vi "Main.vi"() -> ()   [LabVIEW 2025]
doc: "This simple VI control few elements of a Nikon Ti2 microscope.\nAny kind of supplementary element can be controlled with a new event type (flurorescence cube turret for example)"
uses:
  Controls/Presets.ctl
panel:
  in  "Step size (mm?)":dbl
  in  "Move Y+":bool
  in  "Move Y-":bool
  in  "Move X-":bool
  in  "Move X+":bool
  out "XY stage cluster":T1
  out "PFS cluster":T2
  in  "Presets":T3=2 items=["1- Bino - Brightfield"=1, "2- Bino - Fluo"=2, "3- Right - Brightfield"=3, "4- Right - Fluo"=4, "5- Left"=5]
  in  "Cluster commandes":T4={"Dia lamp"=TRUE, "Dia lamp intensity"=1689.1304347826087, "Objective"=2, "Light path"=2, "Z pos (µm)"=335593, "Filter wheel 2"=2, "Filter wheel 1"=2, "Shutter 2"=TRUE, "Shutter 1"=TRUE} {"Filter wheel 1" items=["1"=1, "2"=2, "3"=3, "4"=4, "5"=5, "6"=6]; "Filter wheel 2" items=["1"=1, "2"=2, "3"=3, "4"=4, "5"=5, "6"=6]; "Z pos (µm)" min=0 max=990000 step=100 scale=0.0..990000.0; "Light path" items=["1- Eyepiece"=1, "2- Right"=2, "3- Left + Eyepiece"=3, "4- Left"=4]; "Objective" items=["1- PLAN APO 100X 1,45 Oil"=1, "2- Empty"=2, "3- Empty"=3, "4- Empty"=4, "5- Empty"=5, "6- Empty"=6]; "Dia lamp intensity" scale=0.0..2100.0}
  out "Cluster µscope":T5
  in  "stop":bool
  in  "NikonTi2AxLib.INikonTi2AxMicroscope":refnum<k7>
  out "error out":errorcluster={"status"=TRUE, "code"=-9, "source"="Exception occured in Nikon.Ti2.Microscope.1: Failed in 231026_NikonTi2_Indicators_v2.vi"} caption="sortie d'erreur"
  in  "error in":errorcluster caption="entrée d'erreur"
  # "XY Stage"
  # "Perfect\nFocus\nSystem"
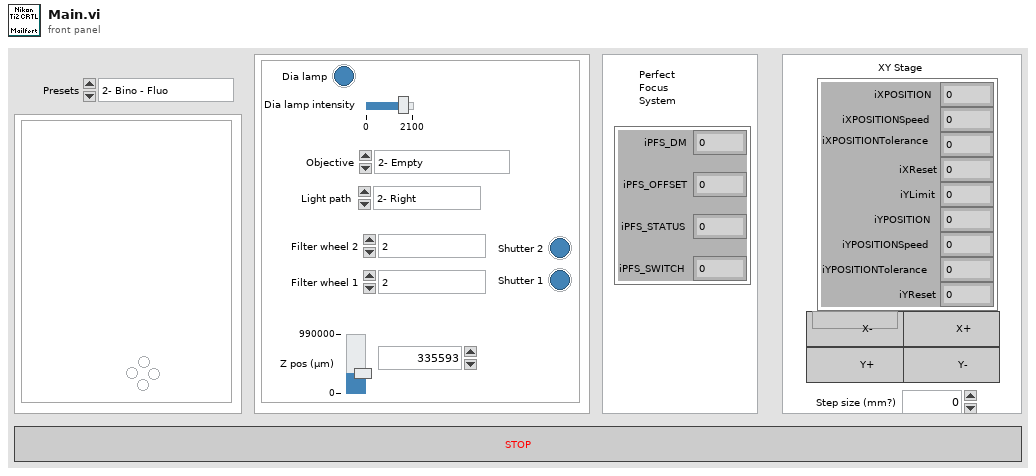
[diagram p1: front panel]
types:
  T1 = cluster{"iXPOSITION":i32, "iXPOSITIONSpeed":i32, "iXPOSITIONTolerance":i32, "iXReset":i32, "iYLimit":i32, "iYPOSITION":i32, "iYPOSITIONSpeed":i32, "iYPOSITIONTolerance":i32, "iYReset":i32}
  T2 = cluster{"iPFS_DM":i32, "iPFS_OFFSET":i32, "iPFS_STATUS":i32, "iPFS_SWITCH":i32}
  T3 = typedef "Presets.ctl" = u8
  T4 = cluster{"Dia lamp":bool, "Dia lamp intensity":dbl, "Objective":i32, "Light path":u32, "Z pos (µm)":i32, "Filter wheel 2":u32, "Filter wheel 1":u32, "Shutter 2":bool, "Shutter 1":bool}
  T5 = cluster{"Eyepiece":bool, "Right":bool, "Left + Eyepiece":bool, "Left":bool}
  T6 = cluster{"iNOSEPIECE":i32, "iLIGHTPATH":i32, "iDIA_LAMP_Switch":i32, "iDIA_LAMP_Pos":i32, "iZPOSITION":i32, "iPFS_SWITCH":i32, "iPFS_STATUS":i32, "iPFS_OFFSET":i32, "iTURRET2POS":i32, "Value":i32, "iTURRET1POS":i32, "Value":i32, "iOPTZOOM":i32}
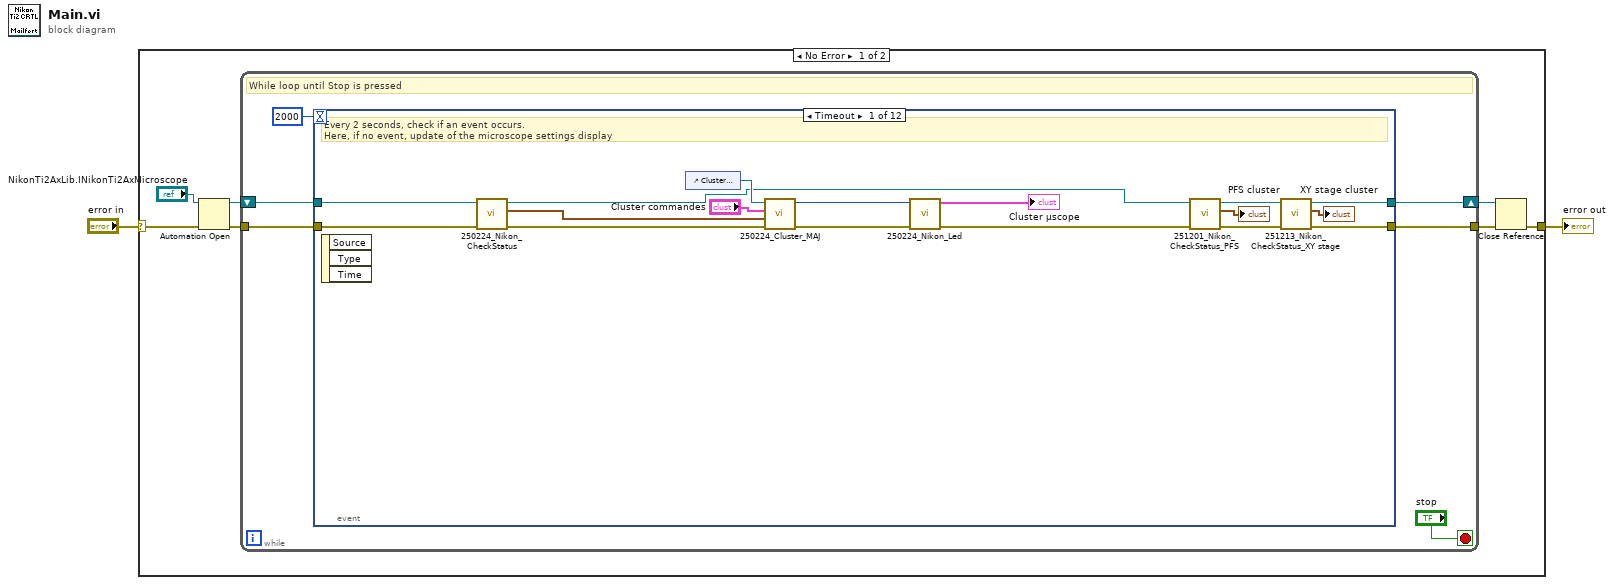
[diagram p0: block diagram]
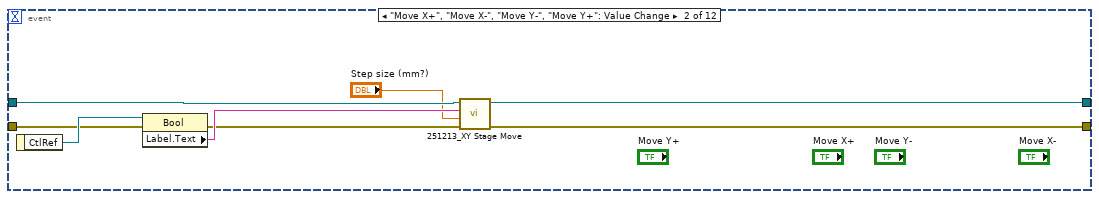
[diagram p2: hidden frame]
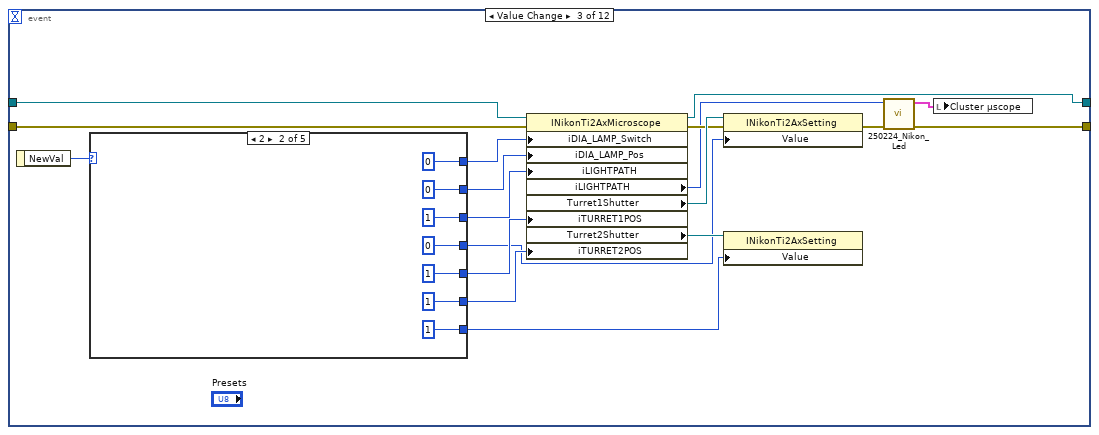
[diagram p3: hidden frame]
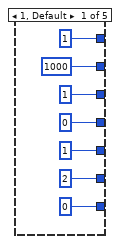
[diagram p4: hidden frame]
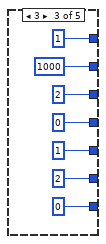
[diagram p5: hidden frame]
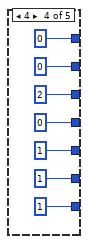
[diagram p6: hidden frame]
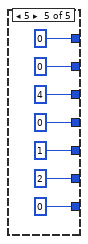
[diagram p7: hidden frame]
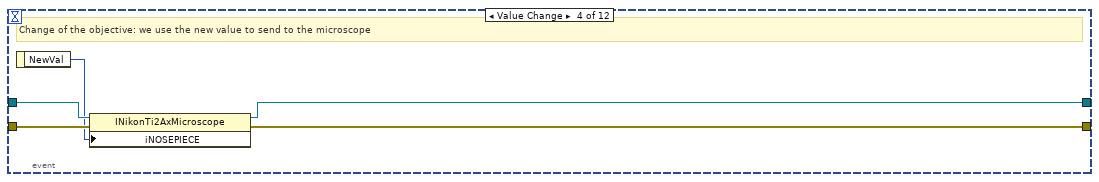
[diagram p8: hidden frame]
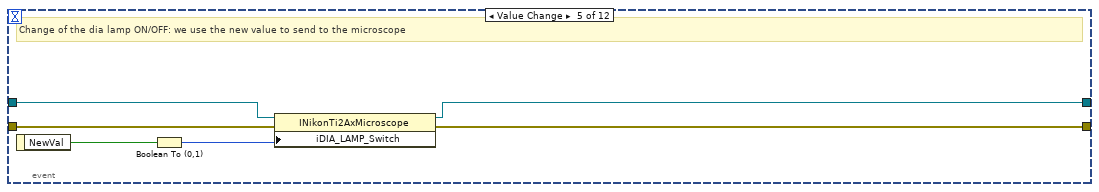
[diagram p9: hidden frame]
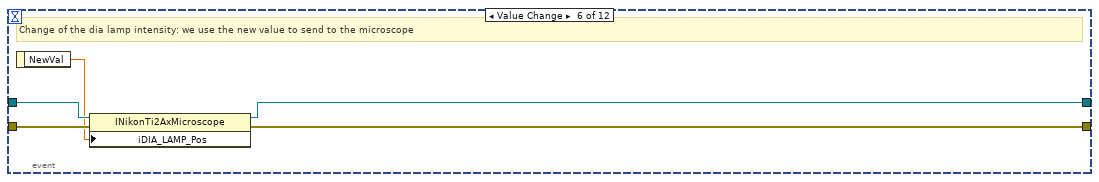
[diagram p10: hidden frame]
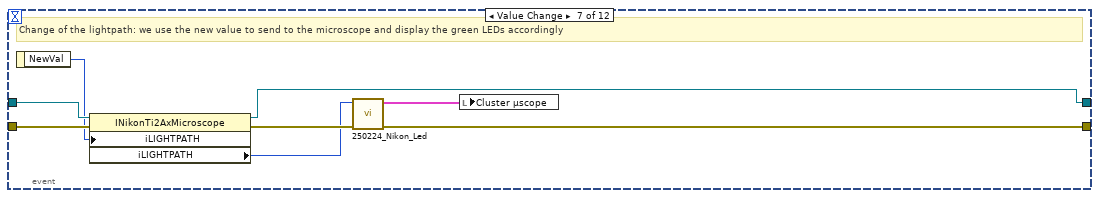
[diagram p11: hidden frame]
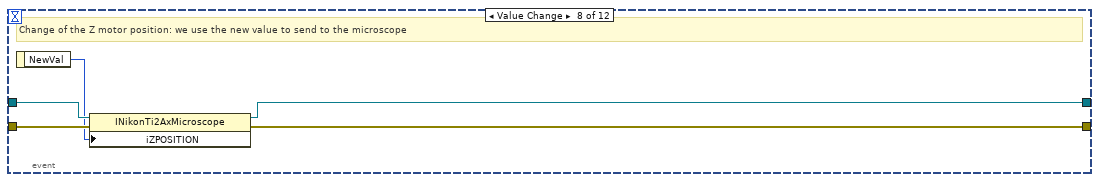
[diagram p12: hidden frame]
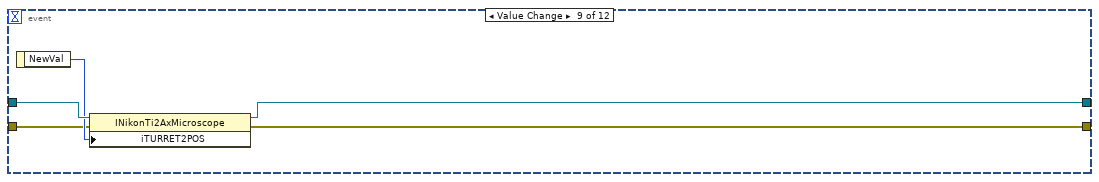
[diagram p13: hidden frame]
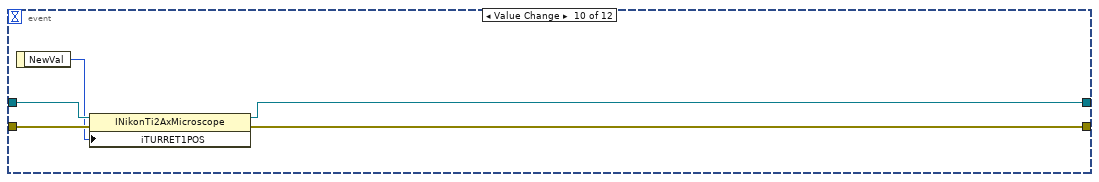
[diagram p14: hidden frame]
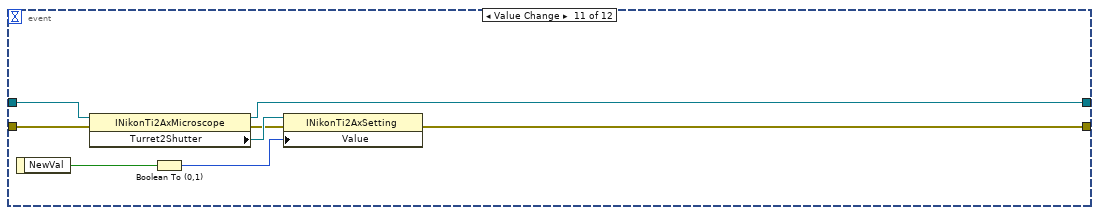
[diagram p15: hidden frame]
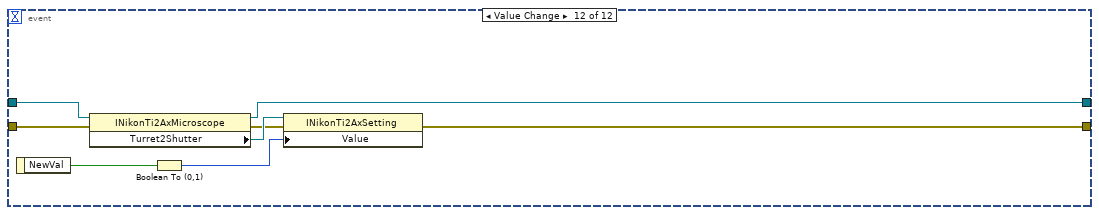
[diagram p16: hidden frame]
diagram:
  n1 = case shown="No Error" "error in" {
    selector: "error in" -> [w8 w149]
    tunnel: [w9 w149] -> w1
    frame No Error {
      n2 = Automation Open(error in (no error)=w8, Automation Refnum="NikonTi2AxLib.INikonTi2AxMicroscope") -> (Automation Refnum=w3:refnum<k7>, error out=w4:errorcluster)  [unwired: 2 in]
      n3 = while {
        shift-right: [w11] -> w7
        shift-left: w3 -> [w12]
        tunnel: w4 -> [w15]
        tunnel: [w10] -> w6
        stop <- "stop" stop-if-true
        # "While loop until Stop is pressed"
        n4 = event shown="[0] Timeout" {
          selector: _ -> [_ _ _ _ _ _ _ _ _ _ _ _]
          dyn-events: _ -> [_ _ _ _ _ _ _ _ _ _ _ _]
          timeout: 2000 -> [_ _ _ _ _ _ _ _ _ _ _ _]
          tunnel: [w19 w33 w57 w95 w101 w106 w114 w120 w124 w128 w135 w143] -> w10
          tunnel: w15 -> [w32 w39 w52 w97 w103 w108 w115 w121 w125 w131 w140 w148]
          tunnel: w12 -> [w31 w36 w53 w98 w104 w109 w116 w122 w127 w132 w139 w147]
          tunnel: [w20 w34 w41 w96 w102 w107 w117 w118 w123 w129 w136 w144] -> w11
          event Timeout {
            # "Every 2 seconds, check if an event occurs.\nHere, if no event, update of the microscope settings display"
            n5 = event-data() -> ()  [unwired: 1 in, 3 out]
            n6 = call "250224_Nikon_CheckStatus.vi"("error in"=w32, "NikonTi2AxLib.INikonTi2AxMicroscope"=w31) -> ("error out"=w29:errorcluster, "Nikon Cluster"=w22:T6, "reference out"=w24:refnum<k7>)  [unwired: 7 in]
            n7 = control-ref of="Cluster commandes"() -> (w26:refnum<vi>)
            n8 = call "250224_Cluster_MAJ.vi"("error in (no error)"=w29, "Nikon Cluster"=w22, 10:"Cluster commandes"="Cluster commandes", 11:"Cluster commandes"=w26) -> ("error out"=w28:errorcluster, "iLIGHTPATH"=w27:i32)  [unwired: 6 in]
            n9 = call "250224_Nikon_Led.vi"("error in"=w28, "Light path"=w27) -> ("error out"=w25:errorcluster, "Cluster µscope"=→"Cluster µscope":T5)  [unwired: 8 in]
            n10 = call "251201_Nikon_CheckStatus_PFS.vi"("error in"=w25, "NikonTi2AxLib.INikonTi2AxMicroscope"=w24) -> ("error out"=w18:errorcluster, "PFS cluster"=→"PFS cluster":T2, "reference out"=w21:refnum<k7>)  [unwired: 7 in]
            n11 = call "251213_Nikon_CheckStatus_XY stage.vi"("error in"=w18, "NikonTi2AxLib.INikonTi2AxMicroscope"=w21) -> ("error out"=w19:errorcluster, "XY stage cluster"=→"XY stage cluster":T1, "reference out"=w20:refnum<k7>)  [unwired: 7 in]
          }
          event "Move X+", "Move X-", "Move Y-", "Move Y+": Value Change {
            n12 = event-data() -> ("CtlRef"=w40:refnum<vi>)  [unwired: 1 in]
            n13 = property class="Bool"(reference=w40, error in=w39) -> (error out=w37:errorcluster, "Label.Text"=w38:string)  [unwired: 1 out]
            n14 = call "251213_XY Stage Move.vi"("error in (no error)"=w37, "Step size (mm?)"="Step size (mm?)", "Label.Text"=w38, "Automation Refnum in"=w36) -> ("error out"=w33:errorcluster, "Automation Refnum out"=w34:refnum<k7>)  [unwired: 6 in]
          }
          event Value Change {
            n15 = event-data() -> ("NewVal"=w56:T3)  [unwired: 1 in]
            n16 = case shown="2" w56 {
              tunnel: [1 0 1 0 0] -> w48
              tunnel: [1000 0 1000 0 0] -> w47
              tunnel: [1 ("iLIGHTPATH") 1 ("iLIGHTPATH") 2 ("iLIGHTPATH") 2 ("iLIGHTPATH") 4 ("iLIGHTPATH")] -> w46
              tunnel: [1 ("iLIGHTPATH") 1 ("iLIGHTPATH") 1 ("iLIGHTPATH") 1 ("iLIGHTPATH") 1 ("iLIGHTPATH")] -> w45
              tunnel: [2 ("iLIGHTPATH") 1 ("iLIGHTPATH") 2 ("iLIGHTPATH") 1 ("iLIGHTPATH") 2 ("iLIGHTPATH")] -> w44
              tunnel: [0 ("iLIGHTPATH") 0 ("iLIGHTPATH") 0 ("iLIGHTPATH") 0 ("iLIGHTPATH") 0 ("iLIGHTPATH")] -> w43
              tunnel: [0 ("iLIGHTPATH") 1 ("iLIGHTPATH") 0 ("iLIGHTPATH") 1 ("iLIGHTPATH") 0 ("iLIGHTPATH")] -> w42
              frame 1, Default {
              }
              frame 2 {
              }
              frame 3 {
              }
              frame 4 {
              }
              frame 5 {
              }
            }
            n17 = property class="INikonTi2AxMicroscope"(reference=w53, error in=w52, "iDIA_LAMP_Switch"=w48, "iDIA_LAMP_Pos"=w47, "iLIGHTPATH"=w46, "iTURRET1POS"=w45, "iTURRET2POS"=w44) -> (reference out=w41:refnum<k7>, error out=w51:errorcluster, "iLIGHTPATH"=w49:i32, "Turret1Shutter"=w55:refnum<k7>, "Turret2Shutter"=w54:refnum<k7>)
            n18 = property class="INikonTi2AxSetting"(reference=w55, error in=w51, "Value"=w43) -> (error out=w50:errorcluster)  [unwired: 1 out]
            n19 = property class="INikonTi2AxSetting"(reference=w54, "Value"=w42) -> ()  [unwired: 1 in, 2 out]
            n20 = call "250224_Nikon_Led.vi"("error in"=w50, "Light path"=w49) -> ("error out"=w57:errorcluster, "Cluster µscope"=w58:T5)  [unwired: 8 in]
            n21 = local write "Cluster µscope"(w58) -> ()
          }
          event "Cluster commandes.Objective": Value Change {
            # "Change of the objective: we use the new value to send to the microscope"
            n22 = event-data() -> ("NewVal"=w94:i32)  [unwired: 1 in]
            n23 = property class="INikonTi2AxMicroscope"(reference=w98, error in=w97, "iNOSEPIECE"=w94) -> (reference out=w96:refnum<k7>, error out=w95:errorcluster)
          }
          event "Cluster commandes.Dia lamp": Value Change {
            # "Change of the dia lamp ON/OFF: we use the new value to send to the microscope"
            n24 = event-data() -> ("NewVal"=w100:bool)  [unwired: 1 in]
            n25 = Boolean To (0,1)(Boolean=w100) -> (0, 1=w99:i16)
            n26 = property class="INikonTi2AxMicroscope"(reference=w104, error in=w103, "iDIA_LAMP_Switch"=w99) -> (reference out=w102:refnum<k7>, error out=w101:errorcluster)
          }
          event "Cluster commandes.Dia lamp intensity": Value Change {
            # "Change of the dia lamp intensity: we use the new value to send to the microscope"
            n27 = event-data() -> ("NewVal"=w105:dbl)  [unwired: 1 in]
            n28 = property class="INikonTi2AxMicroscope"(reference=w109, error in=w108, "iDIA_LAMP_Pos"=w105) -> (reference out=w107:refnum<k7>, error out=w106:errorcluster)
          }
          event "Cluster commandes.Light path": Value Change {
            # "Change of the lightpath: we use the new value to send to the microscope and display the green LEDs accordingly"
            n29 = event-data() -> ("NewVal"=w111:u32)  [unwired: 1 in]
            n30 = property class="INikonTi2AxMicroscope"(reference=w116, error in=w115, "iLIGHTPATH"=w111) -> (reference out=w117:refnum<k7>, error out=w113:errorcluster, "iLIGHTPATH"=w112:i32)
            n31 = call "250224_Nikon_Led.vi"("error in"=w113, "Light path"=w112) -> ("error out"=w114:errorcluster, "Cluster µscope"=w110:T5)  [unwired: 8 in]
            n32 = local write "Cluster µscope"(w110) -> ()
          }
          event "Cluster commandes.Z pos (µm)": Value Change {
            # "Change of the Z motor position: we use the new value to send to the microscope"
            n33 = event-data() -> ("NewVal"=w119:i32)  [unwired: 1 in]
            n34 = property class="INikonTi2AxMicroscope"(reference=w122, error in=w121, "iZPOSITION"=w119) -> (reference out=w118:refnum<k7>, error out=w120:errorcluster)
          }
          event "Cluster commandes.Filter wheel 2": Value Change {
            n35 = event-data() -> ("NewVal"=w126:u32)  [unwired: 1 in]
            n36 = property class="INikonTi2AxMicroscope"(reference=w127, error in=w125, "iTURRET2POS"=w126) -> (reference out=w123:refnum<k7>, error out=w124:errorcluster)
          }
          event "Cluster commandes.Filter wheel 1": Value Change {
            n37 = event-data() -> ("NewVal"=w130:u32)  [unwired: 1 in]
            n38 = property class="INikonTi2AxMicroscope"(reference=w132, error in=w131, "iTURRET1POS"=w130) -> (reference out=w129:refnum<k7>, error out=w128:errorcluster)
          }
          event "Cluster commandes.Shutter 2": Value Change {
            n39 = event-data() -> ("NewVal"=w134:bool)  [unwired: 1 in]
            n40 = property class="INikonTi2AxMicroscope"(reference=w139, error in=w140) -> (reference out=w136:refnum<k7>, error out=w137:errorcluster, "Turret2Shutter"=w138:refnum<k7>)
            n41 = Boolean To (0,1)(Boolean=w134) -> (0, 1=w133:i16)
            n42 = property class="INikonTi2AxSetting"(reference=w138, error in=w137, "Value"=w133) -> (error out=w135:errorcluster)  [unwired: 1 out]
          }
          event "Cluster commandes.Shutter 1": Value Change {
            n43 = event-data() -> ("NewVal"=w142:bool)  [unwired: 1 in]
            n44 = property class="INikonTi2AxMicroscope"(reference=w147, error in=w148) -> (reference out=w144:refnum<k7>, error out=w145:errorcluster, "Turret2Shutter"=w146:refnum<k7>)
            n45 = Boolean To (0,1)(Boolean=w142) -> (0, 1=w141:i16)
            n46 = property class="INikonTi2AxSetting"(reference=w146, error in=w145, "Value"=w141) -> (error out=w143:errorcluster)  [unwired: 1 out]
          }
        }
      }
      n47 = Close Reference(reference=w7, error in (no error)=w6) -> (error out=w9:errorcluster)
    }
    frame Error {
    }
  }
  "error out" <- w1
